vi "Maintain INI File RW.vi"(8 "ErrorIn":errorcluster, 10 "Action":enum16{"Load", "Save"}(ring), 11 "Path":path) -> (0 "ErrorOut":errorcluster)   [LabVIEW 2015]
uses:
  <vilib>/Utility/config.llb/NI_LVConfig.lvlib
  <vilib>/Utility/config.llb/Read Key (I32).vi
  <vilib>/Utility/config.llb/Read Key (Double).vi
  <vilib>/Utility/config.llb/Read Key (U32).vi
  VishayPG 254/Software/Code/INI Struct.ctl
  <vilib>/Utility/config.llb/Read Key (String).vi
  <vilib>/Utility/config.llb/Write Key (Double).vi
  <vilib>/Utility/config.llb/Read Key (Boolean).vi
  <vilib>/Utility/config.llb/Write Key (Boolean).vi
  <vilib>/Utility/config.llb/Write Key (U32).vi
  Controls/Maintain_Struct.ctl
panel:
  out "PanelData_Out":T1
  in  "PanelData_In":T1
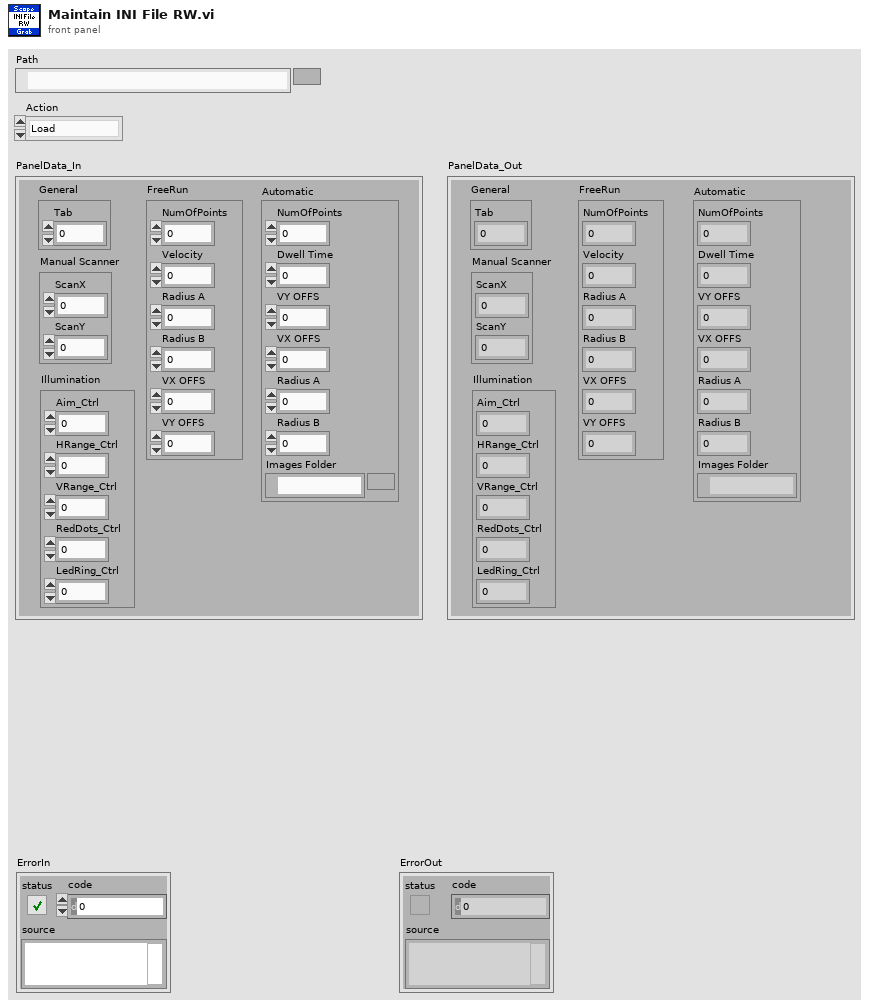
[diagram p1: front panel]
types:
  T1 = typedef "Maintain_Struct.ctl" = cluster{"General":cluster{"Tab":u32}, "Manual Scanner":cluster{"ScanX":dbl, "ScanY":dbl}, "Illumination":cluster{"Aim_Ctrl":dbl, "HRange_Ctrl":dbl, "VRange_Ctrl":dbl, "RedDots_Ctrl":dbl, "LedRing_Ctrl":dbl}, "FreeRun":cluster{"NumOfPoints":u16, "Velocity":dbl, "Radius A":dbl, "Radius B":dbl, "VX OFFS":fxp<+/-,20,5>, "VY OFFS":fxp<+/-,20,5>}, "Automatic":cluster{"NumOfPoints":u16, "Dwell Time":dbl, "VY OFFS":fxp<+/-,20,5>, "VX OFFS":fxp<+/-,20,5>, "Radius A":dbl, "Radius B":dbl, "Images Folder":path}}
  T2 = typedef "NI_LVConfig.lvlib/Config Data RefNum.ctl" = refnum<k1>
  T3 = typedef "INI Struct.ctl" = cluster{"First CH":cluster{"Channel":i32, "Scale":dbl, "Position":dbl, "Coupling":enum16{"AC", "DC"}, "Atten":dbl, "Impedance":enum16{"1 MOhm", "50 Ohm"}}, "Second CH":cluster{"Channel":i32, "Scale":dbl, "Position":dbl, "Coupling":enum16{"AC", "DC"}, "Atten":dbl, "Impedance":enum16{"1 MOhm", "50 Ohm"}}, "Horizontal":cluster{"Scale":dbl, "Position":dbl, "NumOfPoints":u32}, "Trigger":cluster{"Source":enum16{"CH1", "CH2", "CH3", "CH4"}, "Coupling":enum16{"AC", "DC", "LF Reject"}, "Slope":enum16{"Positive", "Negative", "Either", "Altrnate"}, "Level":dbl, "Filter":enum16{"Off", "HP Filter", "LP Filter"}}, "General":cluster{"Scope Address":string, "Operator Name":string, "Project":string, "Product Name":string, "Sample Name":string, "Comments":string, "Simulation Mode":bool, "Result Path":string}}
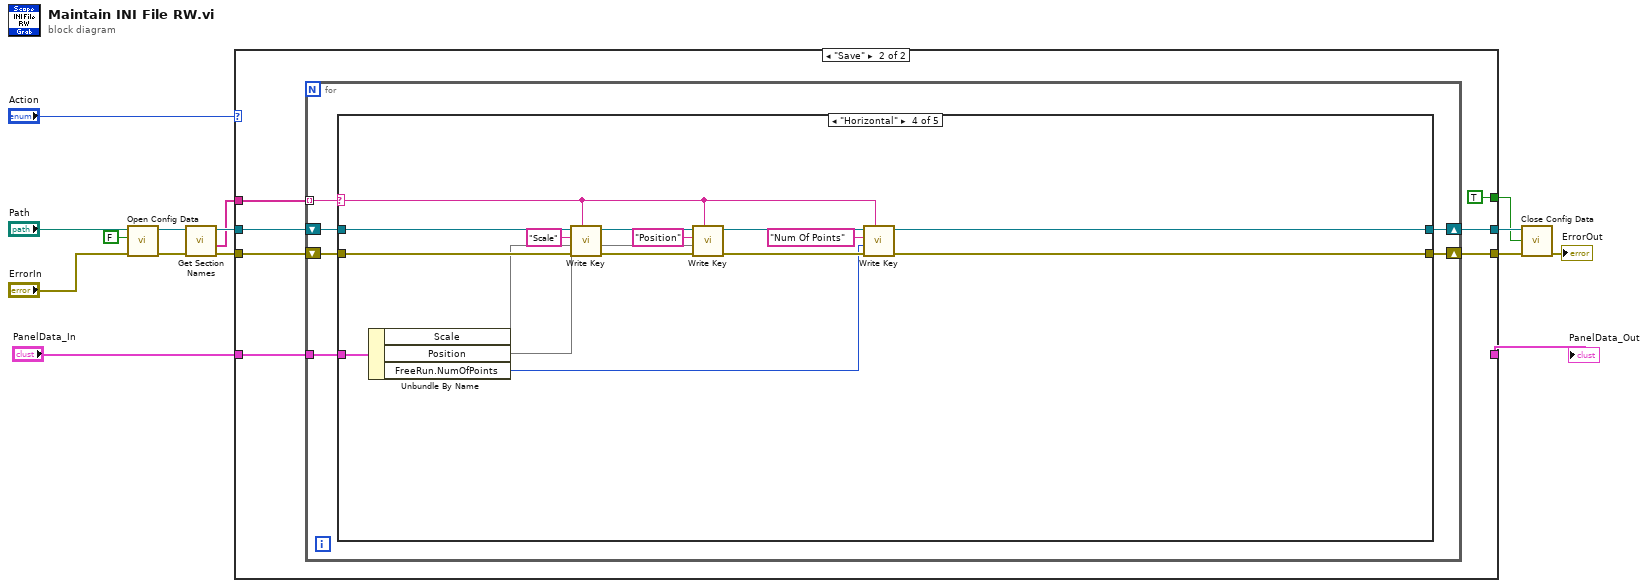
[diagram p0: block diagram]
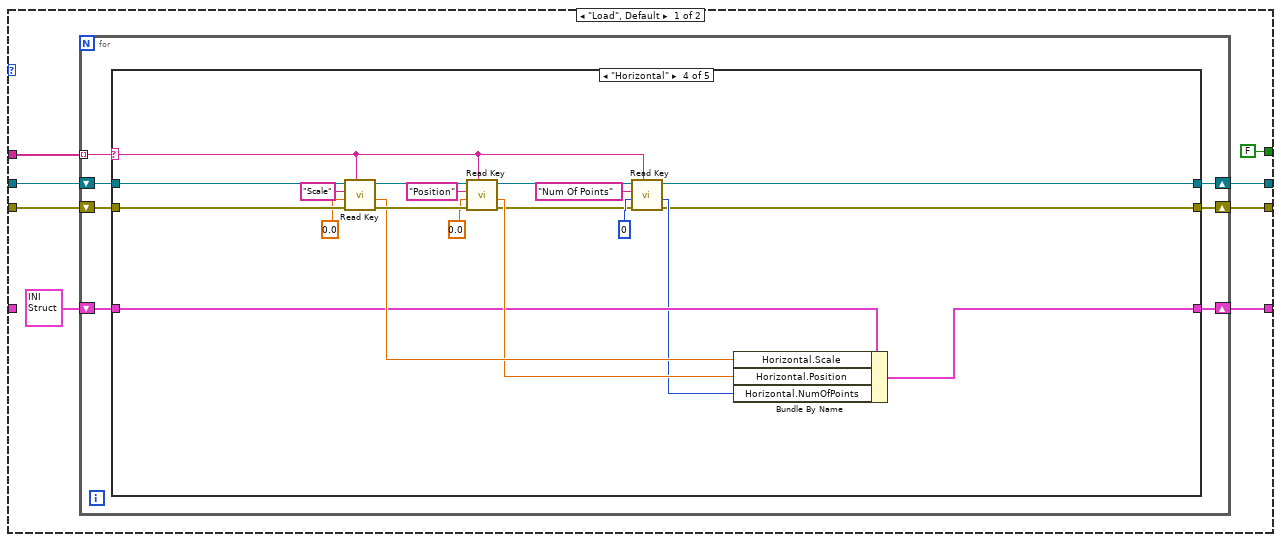
[diagram p2: hidden frame]
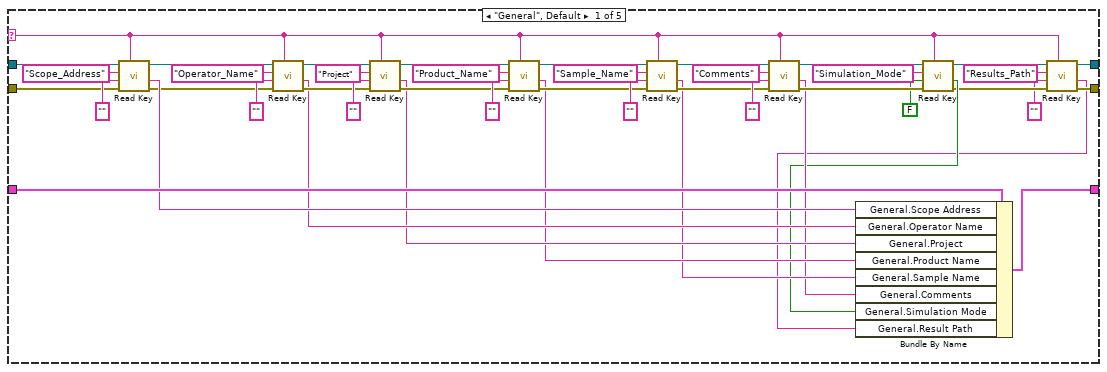
[diagram p3: hidden frame]
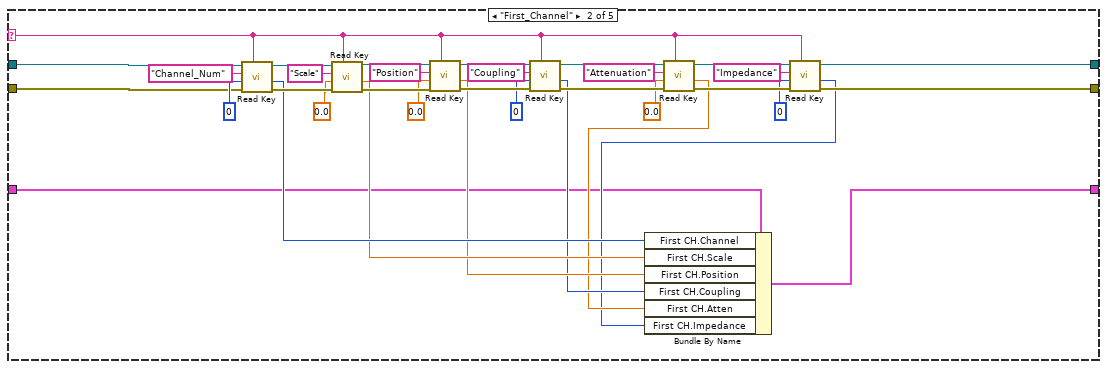
[diagram p4: hidden frame]
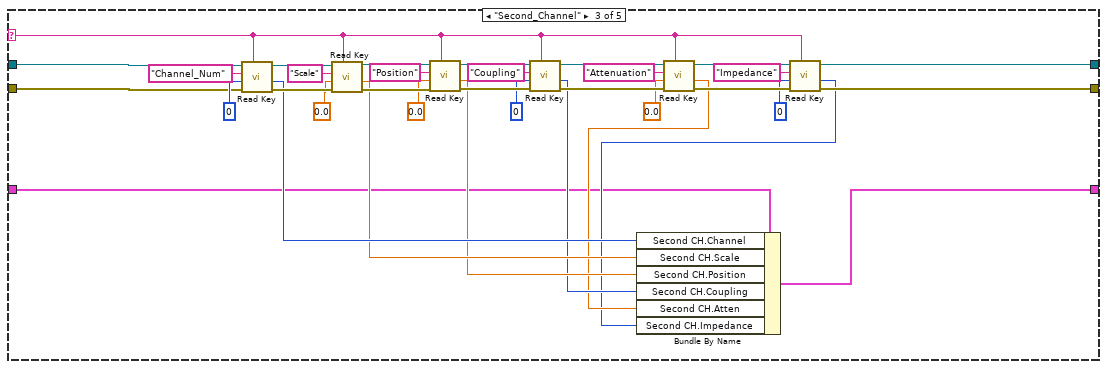
[diagram p5: hidden frame]
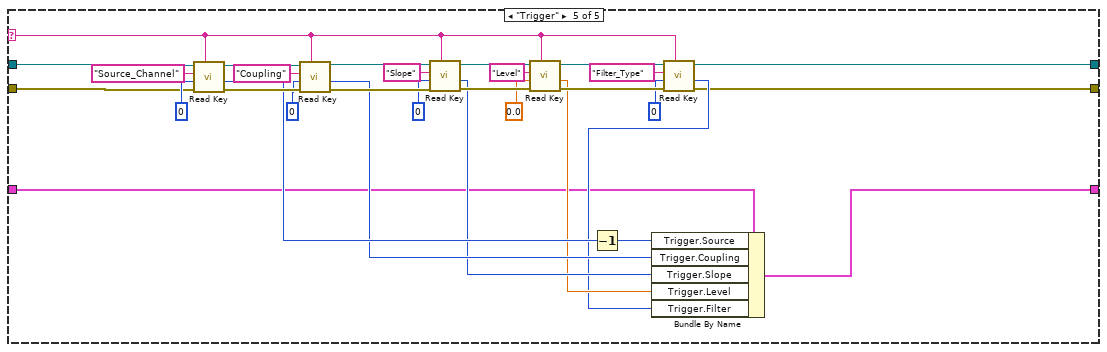
[diagram p6: hidden frame]
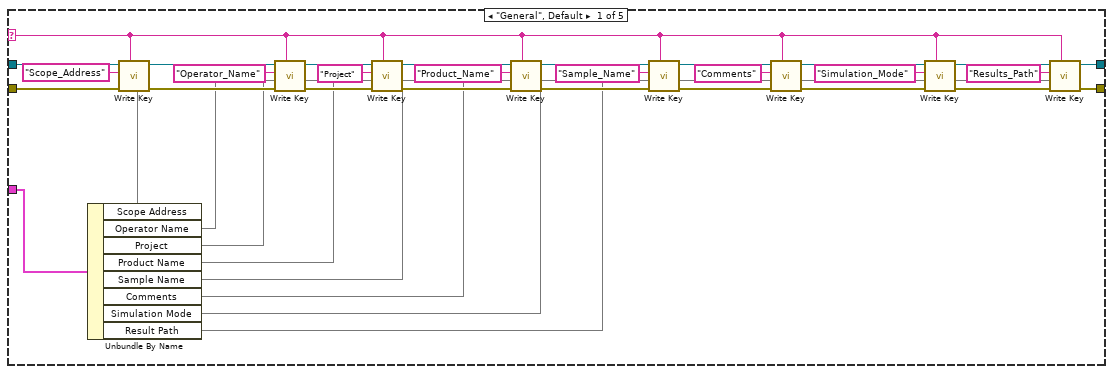
[diagram p7: hidden frame]
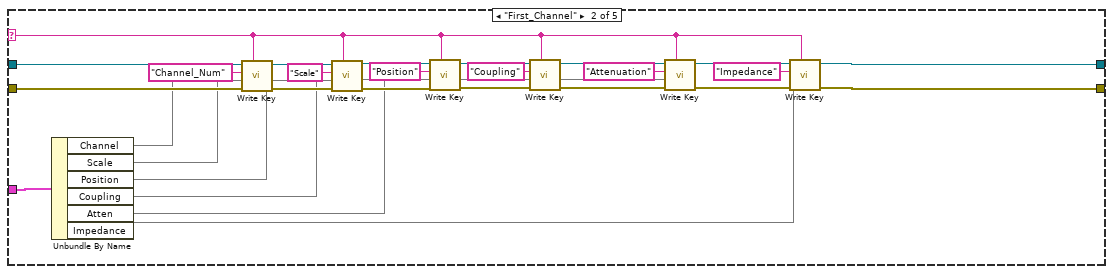
[diagram p8: hidden frame]
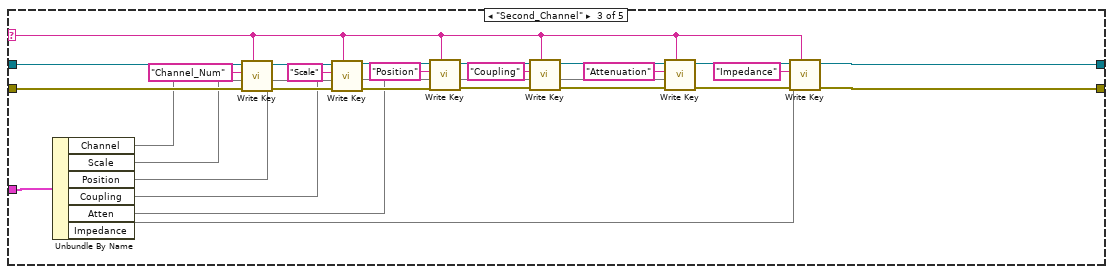
[diagram p9: hidden frame]
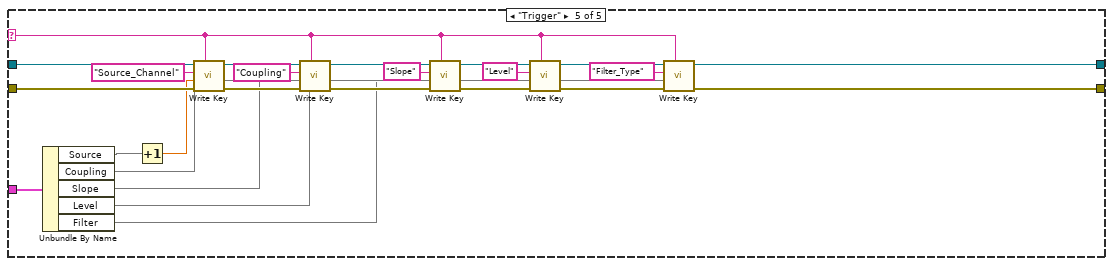
[diagram p10: hidden frame]
diagram:
  n1 = call <vilib>:"Open Config Data.vi"("error in (no error)"="ErrorIn", "create file if necessary (T)"=FALSE, "configuration file path"="Path") -> ("error out"=w10:errorcluster, "refnum"=w9:T2)  [unwired: 6 in, 1 out]
  n2 = call <vilib>:"Get Section Names.vi"("error in (no error)"=w10, "refnum"=w9) -> ("error out"=w7:errorcluster, "section names"=w6:string[], "refnum out"=w8:T2)  [unwired: 7 in]
  n3 = case shown="\"Save\"" "Action" {
    tunnel: [w23 w203] -> w15
    tunnel: [w22 w202] -> w14
    tunnel: w8 -> [w21 w201]
    tunnel: w7 -> [w20 w200]
    tunnel: w6 -> [w19 w199]
    tunnel: [w18 _] -> w1
    tunnel: "PanelData_In" -> [_ w198]
    tunnel: [FALSE TRUE] -> w4
    frame "Load", Default {
      n4 = for {
        shift-right: [w30] -> w22
        shift-left: w21 -> [w29]
        shift-right: [w24] -> w23
        shift-left: w20 -> [w28]
        tunnel: w19 -> [w27] mode=indexing
        shift-right: [w25] -> w18
        shift-left: T3 {"First CH"={"Channel"=0, "Scale"=0.0, "Position"=0.0, "Coupling"=enum."AC", "Atten"=0.0, "Impedance"=enum."1 MOhm"}, "Second CH"={"Channel"=0, "Scale"=0.0, "Position"=0.0, "Coupling"=enum."AC", "Atten"=0.0, "Impedance"=enum."1 MOhm"}, "Horizontal"={"Scale"=0.0, "Position"=0.0, "NumOfPoints"=0}, "Trigger"={"Source"=enum."CH1", "Coupling"=enum."AC", "Slope"=enum."Positive", "Level"=0.0, "Filter"=enum."Off"}, "General"={"Scope Address"="", "Operator Name"="", "Project"="", "Product Name"="", "Sample Name"="", "Comments"="", "Simulation Mode"=FALSE, "Result Path"=""}} ("DataOut") -> [w26]
        n5 = case shown="\"Horizontal\"" w27 {
          selector: w27 -> [w35 w76 w111 w149 w169]
          tunnel: [w34 w93 w128 w146 w167] -> w30
          tunnel: w29 -> [w72 w77 w112 w155 w170]
          tunnel: w28 -> [w73 w78 w113 w156 w171]
          tunnel: w26 -> [w71 w80 w115 w158 w173]
          tunnel: [w69 w79 w114 w157 w172] -> w25
          tunnel: [w33 w94 w129 w147 w168] -> w24
          frame "General", Default {
            n6 = call-poly <vilib>:"Read Key.vi"("section"=w35, "error in (no error)"=w73, "default value"="", "key"="Scope_Address", "refnum"=w72) -> ("error out"=w66:errorcluster, "value"=w70:string, "refnum out"=w65:T2)  [unwired: 3 in, 1 out]
            n7 = call-poly <vilib>:"Read Key.vi"("section"=w35, "error in (no error)"=w66, "default value"="", "key"="Operator_Name", "refnum"=w65) -> ("error out"=w62:errorcluster, "value"=w45:string, "refnum out"=w61:T2)  [unwired: 3 in, 1 out]
            n8 = call-poly <vilib>:"Read Key.vi"("section"=w35, "error in (no error)"=w62, "default value"="", "key"="Project", "refnum"=w61) -> ("error out"=w58:errorcluster, "value"=w44:string, "refnum out"=w57:T2)  [unwired: 3 in, 1 out]
            n9 = call-poly <vilib>:"Read Key.vi"("section"=w35, "error in (no error)"=w58, "default value"="", "key"="Product_Name", "refnum"=w57) -> ("error out"=w54:errorcluster, "value"=w43:string, "refnum out"=w53:T2)  [unwired: 3 in, 1 out]
            n10 = call-poly <vilib>:"Read Key.vi"("section"=w35, "error in (no error)"=w54, "default value"="", "key"="Sample_Name", "refnum"=w53) -> ("error out"=w50:errorcluster, "value"=w42:string, "refnum out"=w49:T2)  [unwired: 3 in, 1 out]
            n11 = call-poly <vilib>:"Read Key.vi"("section"=w35, "error in (no error)"=w50, "default value"="", "key"="Comments", "refnum"=w49) -> ("error out"=w47:errorcluster, "value"=w41:string, "refnum out"=w46:T2)  [unwired: 3 in, 1 out]
            n12 = call-poly <vilib>:"Read Key.vi"("section"=w35, "error in (no error)"=w47, "default value"=FALSE, "key"="Simulation_Mode", "refnum"=w46) -> ("error out"=w38:errorcluster, "value"=w39:bool, "refnum out"=w36:T2)  [unwired: 3 in, 1 out]
            n13 = call-poly <vilib>:"Read Key.vi"("section"=w35, "error in (no error)"=w38, "default value"="", "key"="Results_Path", "refnum"=w36) -> ("error out"=w33:errorcluster, "value"=w31:string, "refnum out"=w34:T2)  [unwired: 3 in, 1 out]
            n14 = Bundle By Name(cluster=w71, "General.Scope Address"=w70, "General.Operator Name"=w45, "General.Project"=w44, "General.Product Name"=w43, "General.Sample Name"=w42, "General.Comments"=w41, "General.Simulation Mode"=w39, "General.Result Path"=w31) -> (w69:T3)
          }
          frame "First_Channel" {
            n15 = call-poly <vilib>:"Read Key.vi"("section"=w76, "error in (no error)"=w78, "default value"=0, "key"="Channel_Num", "refnum"=w77) -> ("error out"=w104:errorcluster, "value"=w92:i32, "refnum out"=w109:T2)  [unwired: 3 in, 1 out]
            n16 = call-poly <vilib>:"Read Key.vi"("section"=w76, "error in (no error)"=w104, "default value"=0.0, "key"="Scale", "refnum"=w109) -> ("error out"=w103:errorcluster, "value"=w85:dbl, "refnum out"=w105:T2)  [unwired: 3 in, 1 out]
            n17 = call-poly <vilib>:"Read Key.vi"("section"=w76, "error in (no error)"=w103, "default value"=0.0, "key"="Position", "refnum"=w105) -> ("error out"=w102:errorcluster, "value"=w84:dbl, "refnum out"=w106:T2)  [unwired: 3 in, 1 out]
            n18 = call-poly <vilib>:"Read Key.vi"("section"=w76, "error in (no error)"=w102, "default value"=u16 0, "key"="Coupling", "refnum"=w106) -> ("error out"=w101:errorcluster, "value"=w83:u32, "refnum out"=w107:T2)  [unwired: 3 in, 1 out]
            n19 = call-poly <vilib>:"Read Key.vi"("section"=w76, "error in (no error)"=w101, "default value"=0.0, "key"="Attenuation", "refnum"=w107) -> ("error out"=w100:errorcluster, "value"=w82:dbl, "refnum out"=w108:T2)  [unwired: 3 in, 1 out]
            n20 = call-poly <vilib>:"Read Key.vi"("section"=w76, "error in (no error)"=w100, "default value"=u16 0, "key"="Impedance", "refnum"=w108) -> ("error out"=w94:errorcluster, "value"=w81:u32, "refnum out"=w93:T2)  [unwired: 3 in, 1 out]
            n21 = Bundle By Name(cluster=w80, "First CH.Channel"=w92, "First CH.Scale"=w85, "First CH.Position"=w84, "First CH.Coupling"=w83, "First CH.Atten"=w82, "First CH.Impedance"=w81) -> (w79:T3)
          }
          frame "Second_Channel" {
            n22 = call-poly <vilib>:"Read Key.vi"("section"=w111, "error in (no error)"=w113, "default value"=0, "key"="Channel_Num", "refnum"=w112) -> ("error out"=w139:errorcluster, "value"=w127:i32, "refnum out"=w144:T2)  [unwired: 3 in, 1 out]
            n23 = call-poly <vilib>:"Read Key.vi"("section"=w111, "error in (no error)"=w139, "default value"=0.0, "key"="Scale", "refnum"=w144) -> ("error out"=w138:errorcluster, "value"=w120:dbl, "refnum out"=w140:T2)  [unwired: 3 in, 1 out]
            n24 = call-poly <vilib>:"Read Key.vi"("section"=w111, "error in (no error)"=w138, "default value"=0.0, "key"="Position", "refnum"=w140) -> ("error out"=w137:errorcluster, "value"=w119:dbl, "refnum out"=w141:T2)  [unwired: 3 in, 1 out]
            n25 = call-poly <vilib>:"Read Key.vi"("section"=w111, "error in (no error)"=w137, "default value"=u16 0, "key"="Coupling", "refnum"=w141) -> ("error out"=w136:errorcluster, "value"=w118:u32, "refnum out"=w142:T2)  [unwired: 3 in, 1 out]
            n26 = call-poly <vilib>:"Read Key.vi"("section"=w111, "error in (no error)"=w136, "default value"=0.0, "key"="Attenuation", "refnum"=w142) -> ("error out"=w135:errorcluster, "value"=w117:dbl, "refnum out"=w143:T2)  [unwired: 3 in, 1 out]
            n27 = call-poly <vilib>:"Read Key.vi"("section"=w111, "error in (no error)"=w135, "default value"=u16 0, "key"="Impedance", "refnum"=w143) -> ("error out"=w129:errorcluster, "value"=w116:u32, "refnum out"=w128:T2)  [unwired: 3 in, 1 out]
            n28 = Bundle By Name(cluster=w115, "Second CH.Channel"=w127, "Second CH.Scale"=w120, "Second CH.Position"=w119, "Second CH.Coupling"=w118, "Second CH.Atten"=w117, "Second CH.Impedance"=w116) -> (w114:T3)
          }
          frame "Horizontal" {
            n29 = call-poly <vilib>:"Read Key.vi"("section"=w149, "error in (no error)"=w156, "default value"=0.0, "key"="Scale", "refnum"=w155) -> ("error out"=w163:errorcluster, "value"=w161:dbl, "refnum out"=w164:T2)  [unwired: 3 in, 1 out]
            n30 = call-poly <vilib>:"Read Key.vi"("section"=w149, "error in (no error)"=w163, "default value"=0.0, "key"="Position", "refnum"=w164) -> ("error out"=w150:errorcluster, "value"=w159:dbl, "refnum out"=w151:T2)  [unwired: 3 in, 1 out]
            n31 = call-poly <vilib>:"Read Key.vi"("section"=w149, "error in (no error)"=w150, "default value"=u32 0, "key"="Num Of Points", "refnum"=w151) -> ("error out"=w147:errorcluster, "value"=w148:u32, "refnum out"=w146:T2)  [unwired: 3 in, 1 out]
            n32 = Bundle By Name(cluster=w158, "Horizontal.Scale"=w161, "Horizontal.Position"=w159, "Horizontal.NumOfPoints"=w148) -> (w157:T3)
          }
          frame "Trigger" {
            n33 = call-poly <vilib>:"Read Key.vi"("section"=w169, "error in (no error)"=w171, "default value"=0, "key"="Source_Channel", "refnum"=w170) -> ("error out"=w191:errorcluster, "value"=w183:i32, "refnum out"=w195:T2)  [unwired: 3 in, 1 out]
            n34 = call-poly <vilib>:"Read Key.vi"("section"=w169, "error in (no error)"=w191, "default value"=u16 0, "key"="Coupling", "refnum"=w195) -> ("error out"=w190:errorcluster, "value"=w177:u32, "refnum out"=w192:T2)  [unwired: 3 in, 1 out]
            n35 = call-poly <vilib>:"Read Key.vi"("section"=w169, "error in (no error)"=w190, "default value"=u16 0, "key"="Slope", "refnum"=w192) -> ("error out"=w189:errorcluster, "value"=w176:u32, "refnum out"=w193:T2)  [unwired: 3 in, 1 out]
            n36 = call-poly <vilib>:"Read Key.vi"("section"=w169, "error in (no error)"=w189, "default value"=0.0, "key"="Level", "refnum"=w193) -> ("error out"=w188:errorcluster, "value"=w175:dbl, "refnum out"=w194:T2)  [unwired: 3 in, 1 out]
            n37 = Decrement(x=w183) -> (x-1=w166:i32)
            n38 = call-poly <vilib>:"Read Key.vi"("section"=w169, "error in (no error)"=w188, "default value"=u16 0, "key"="Filter_Type", "refnum"=w194) -> ("error out"=w168:errorcluster, "value"=w174:u32, "refnum out"=w167:T2)  [unwired: 3 in, 1 out]
            n39 = Bundle By Name(cluster=w173, "Trigger.Source"=w166, "Trigger.Coupling"=w177, "Trigger.Slope"=w176, "Trigger.Level"=w175, "Trigger.Filter"=w174) -> (w172:T3)
          }
        }
      }
    }
    frame "Save" {
      n40 = for {
        shift-right: [w204] -> w202
        shift-left: w201 -> [w208]
        shift-right: [w209] -> w203
        shift-left: w200 -> [w207]
        tunnel: w199 -> [w206] mode=indexing
        tunnel: w198 -> [w205]
        n41 = case shown="\"Horizontal\"" w206 {
          selector: w206 -> [w211 w253 w281 w305 w327]
          tunnel: [w212 w257 w285 w304 w326] -> w209
          tunnel: w208 -> [w243 w254 w282 w312 w328]
          tunnel: w207 -> [w244 w255 w283 w313 w329]
          tunnel: w205 -> [w242 w252 w280 w311 w324]
          tunnel: [w213 w256 w284 w303 w325] -> w204
          frame "General", Default {
            n42 = Unbundle By Name(w242) -> ("Scope Address"=w223, "Operator Name"=w222, "Project"=w221, "Product Name"=w220, "Sample Name"=w219, "Comments"=w218, "Simulation Mode"=w217, "Result Path"=w210)
            n43 = call-poly <vilib>:"Write Key.vi"("section"=w211, "error in (no error)"=w244, "value"=w223, "key"="Scope_Address", "refnum"=w243) -> ("error out"=w225:errorcluster, "refnum out"=w224:T2)  [unwired: 4 in, 1 out]
            n44 = call-poly <vilib>:"Write Key.vi"("section"=w211, "error in (no error)"=w225, "value"=w222, "key"="Operator_Name", "refnum"=w224) -> ("error out"=w239:errorcluster, "refnum out"=w238:T2)  [unwired: 4 in, 1 out]
            n45 = call-poly <vilib>:"Write Key.vi"("section"=w211, "error in (no error)"=w239, "value"=w221, "key"="Project", "refnum"=w238) -> ("error out"=w236:errorcluster, "refnum out"=w235:T2)  [unwired: 4 in, 1 out]
            n46 = call-poly <vilib>:"Write Key.vi"("section"=w211, "error in (no error)"=w236, "value"=w220, "key"="Product_Name", "refnum"=w235) -> ("error out"=w233:errorcluster, "refnum out"=w232:T2)  [unwired: 4 in, 1 out]
            n47 = call-poly <vilib>:"Write Key.vi"("section"=w211, "error in (no error)"=w233, "value"=w219, "key"="Sample_Name", "refnum"=w232) -> ("error out"=w230:errorcluster, "refnum out"=w229:T2)  [unwired: 4 in, 1 out]
            n48 = call-poly <vilib>:"Write Key.vi"("section"=w211, "error in (no error)"=w230, "value"=w218, "key"="Comments", "refnum"=w229) -> ("error out"=w227:errorcluster, "refnum out"=w226:T2)  [unwired: 4 in, 1 out]
            n49 = call-poly <vilib>:"Write Key.vi"("section"=w211, "error in (no error)"=w227, "value"=w217, "key"="Simulation_Mode", "refnum"=w226) -> ("error out"=w215:errorcluster, "refnum out"=w214:T2)  [unwired: 4 in, 1 out]
            n50 = call-poly <vilib>:"Write Key.vi"("section"=w211, "error in (no error)"=w215, "value"=w210, "key"="Results_Path", "refnum"=w214) -> ("error out"=w212:errorcluster, "refnum out"=w213:T2)  [unwired: 4 in, 1 out]
          }
          frame "First_Channel" {
            n51 = Unbundle By Name(w252) -> ("Channel"=w251, "Scale"=w250, "Position"=w249, "Coupling"=w248, "Atten"=w247, "Impedance"=w246)
            n52 = call-poly <vilib>:"Write Key.vi"("section"=w253, "error in (no error)"=w255, "value"=w251, "key"="Channel_Num", "refnum"=w254) -> ("error out"=w267:errorcluster, "refnum out"=w272:T2)  [unwired: 4 in, 1 out]
            n53 = call-poly <vilib>:"Write Key.vi"("section"=w253, "error in (no error)"=w267, "value"=w250, "key"="Scale", "refnum"=w272) -> ("error out"=w266:errorcluster, "refnum out"=w268:T2)  [unwired: 4 in, 1 out]
            n54 = call-poly <vilib>:"Write Key.vi"("section"=w253, "error in (no error)"=w266, "value"=w249, "key"="Position", "refnum"=w268) -> ("error out"=w265:errorcluster, "refnum out"=w269:T2)  [unwired: 4 in, 1 out]
            n55 = call-poly <vilib>:"Write Key.vi"("section"=w253, "error in (no error)"=w265, "value"=w248, "key"="Coupling", "refnum"=w269) -> ("error out"=w264:errorcluster, "refnum out"=w270:T2)  [unwired: 4 in, 1 out]
            n56 = call-poly <vilib>:"Write Key.vi"("section"=w253, "error in (no error)"=w264, "value"=w247, "key"="Attenuation", "refnum"=w270) -> ("error out"=w263:errorcluster, "refnum out"=w271:T2)  [unwired: 4 in, 1 out]
            n57 = call-poly <vilib>:"Write Key.vi"("section"=w253, "error in (no error)"=w263, "value"=w246, "key"="Impedance", "refnum"=w271) -> ("error out"=w257:errorcluster, "refnum out"=w256:T2)  [unwired: 4 in, 1 out]
          }
          frame "Second_Channel" {
            n58 = Unbundle By Name(w280) -> ("Channel"=w279, "Scale"=w278, "Position"=w277, "Coupling"=w276, "Atten"=w275, "Impedance"=w274)
            n59 = call-poly <vilib>:"Write Key.vi"("section"=w281, "error in (no error)"=w283, "value"=w279, "key"="Channel_Num", "refnum"=w282) -> ("error out"=w295:errorcluster, "refnum out"=w300:T2)  [unwired: 4 in, 1 out]
            n60 = call-poly <vilib>:"Write Key.vi"("section"=w281, "error in (no error)"=w295, "value"=w278, "key"="Scale", "refnum"=w300) -> ("error out"=w294:errorcluster, "refnum out"=w296:T2)  [unwired: 4 in, 1 out]
            n61 = call-poly <vilib>:"Write Key.vi"("section"=w281, "error in (no error)"=w294, "value"=w277, "key"="Position", "refnum"=w296) -> ("error out"=w293:errorcluster, "refnum out"=w297:T2)  [unwired: 4 in, 1 out]
            n62 = call-poly <vilib>:"Write Key.vi"("section"=w281, "error in (no error)"=w293, "value"=w276, "key"="Coupling", "refnum"=w297) -> ("error out"=w292:errorcluster, "refnum out"=w298:T2)  [unwired: 4 in, 1 out]
            n63 = call-poly <vilib>:"Write Key.vi"("section"=w281, "error in (no error)"=w292, "value"=w275, "key"="Attenuation", "refnum"=w298) -> ("error out"=w291:errorcluster, "refnum out"=w299:T2)  [unwired: 4 in, 1 out]
            n64 = call-poly <vilib>:"Write Key.vi"("section"=w281, "error in (no error)"=w291, "value"=w274, "key"="Impedance", "refnum"=w299) -> ("error out"=w285:errorcluster, "refnum out"=w284:T2)  [unwired: 4 in, 1 out]
          }
          frame "Horizontal" {
            n65 = Unbundle By Name(w311) -> ("Scale"=w310, "Position"=w309, "FreeRun.NumOfPoints"=w302:u16)
            n66 = call-poly <vilib>:"Write Key.vi"("section"=w305, "error in (no error)"=w313, "value"=w310, "key"="Scale", "refnum"=w312) -> ("error out"=w315:errorcluster, "refnum out"=w316:T2)  [unwired: 4 in, 1 out]
            n67 = call-poly <vilib>:"Write Key.vi"("section"=w305, "error in (no error)"=w315, "value"=w309, "key"="Position", "refnum"=w316) -> ("error out"=w307:errorcluster, "refnum out"=w306:T2)  [unwired: 4 in, 1 out]
            n68 = call-poly <vilib>:"Write Key.vi"("section"=w305, "error in (no error)"=w307, "value"=w302, "key"="Num Of Points", "refnum"=w306) -> ("error out"=w304:errorcluster, "refnum out"=w303:T2)  [unwired: 4 in, 1 out]
          }
          frame "Trigger" {
            n69 = Unbundle By Name(w324) -> ("Source"=w323, "Coupling"=w322, "Slope"=w321, "Level"=w320, "Filter"=w319)
            n70 = Increment(x=w323) -> (x+1=w318:dbl)
            n71 = call-poly <vilib>:"Write Key.vi"("section"=w327, "error in (no error)"=w329, "value"=w318, "key"="Source_Channel", "refnum"=w328) -> ("error out"=w337:errorcluster, "refnum out"=w341:T2)  [unwired: 4 in, 1 out]
            n72 = call-poly <vilib>:"Write Key.vi"("section"=w327, "error in (no error)"=w337, "value"=w322, "key"="Coupling", "refnum"=w341) -> ("error out"=w336:errorcluster, "refnum out"=w338:T2)  [unwired: 4 in, 1 out]
            n73 = call-poly <vilib>:"Write Key.vi"("section"=w327, "error in (no error)"=w336, "value"=w321, "key"="Slope", "refnum"=w338) -> ("error out"=w335:errorcluster, "refnum out"=w339:T2)  [unwired: 4 in, 1 out]
            n74 = call-poly <vilib>:"Write Key.vi"("section"=w327, "error in (no error)"=w335, "value"=w320, "key"="Level", "refnum"=w339) -> ("error out"=w334:errorcluster, "refnum out"=w340:T2)  [unwired: 4 in, 1 out]
            n75 = call-poly <vilib>:"Write Key.vi"("section"=w327, "error in (no error)"=w334, "value"=w319, "key"="Filter_Type", "refnum"=w340) -> ("error out"=w326:errorcluster, "refnum out"=w325:T2)  [unwired: 4 in, 1 out]
          }
        }
      }
    }
  }
  "PanelData_Out" <- w1
  n76 = call <vilib>:"Close Config Data.vi"("error in (no error)"=w15, "write file if changed (T)"=w4, "refnum"=w14) -> ("error out"=→"ErrorOut":errorcluster)  [unwired: 7 in, 1 out]
